vi "ManualControlL0SumnAdd.vi"(11 "Instrument VISA in":T1={"AWG VISA"="generadorpulsos", "Oscilloscope  VISA "="Oscilloscope", "Integration Board IP"="172.16.7.43", "connection ID"=refnum, "report out"=refnum, "report file path"=path "C:/Documents and Settings/CTA_LAB01/Desktop/L0_Asic/L0 Asic Test Data"}) -> (0 "error out":errorcluster, 3 "Instrument VISA out":T1={"AWG VISA"="generadorpulsos", "Oscilloscope  VISA "="Oscilloscope", "Integration Board IP"="172.16.7.43", "connection ID"=refnum, "report out"=refnum, "report file path"=path "C:/Documents and Settings/CTA_LAB01/Desktop/L0_Asic/L0 Asic Test Data"})   [LabVIEW 2009]
uses:
  <vilib>/Utility/NIReport.llb/NI_report.lvclass
  <vilib>/Utility/NIReport.llb/HTML/NI_HTML.lvclass
  Sum_Abrilader/L0_Sum_Adder Folder/C/Program Files/National Instruments/LabVIEW 2012/instr.lib/Agilent 8000 Series/Public/Configure/Configure Math (Binary Operation).vi
  Sum_Abrilader/L0_Sum_Adder Folder/C/Program Files/National Instruments/LabVIEW 2012/instr.lib/Agilent 8000 Series/Agilent 8000 Series.lvlib
panel:
  in  "error in (no error)":errorcluster
  in  "stop":bool
  in  "Enable 6":bool=TRUE
  in  "Enable 4":bool=TRUE
  in  "Enable 5":bool=TRUE
  in  "Enable 2":bool=TRUE
  in  "Enable 3":bool=TRUE
  in  "Enable 0":bool=TRUE
  in  "Enable 1":bool=TRUE
  in  "Amplitude":dbl=0.1 min=0.05 max=1.0 step=0.05
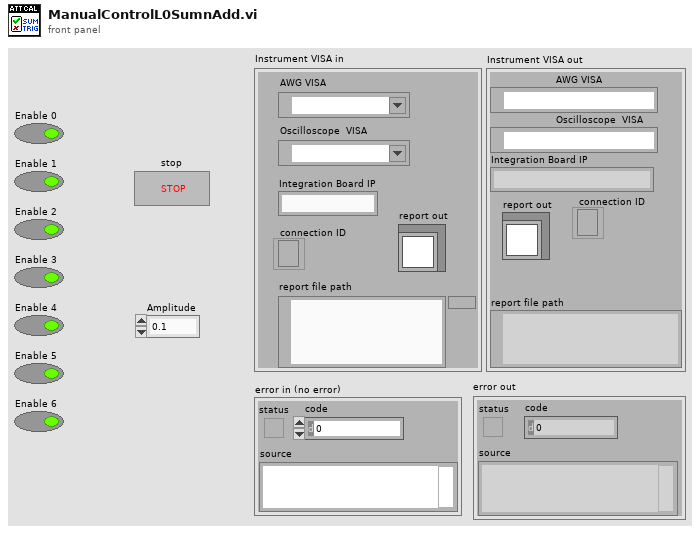
[diagram p1: front panel]
types:
  T1 = cluster{"AWG VISA":refnum<visa-resource-name>, "Oscilloscope  VISA ":refnum<visa-resource-name>, "Integration Board IP":string, "connection ID":refnum<k5>, "report out":refnum<class "NI_report.lvclass">, "report file path":path}
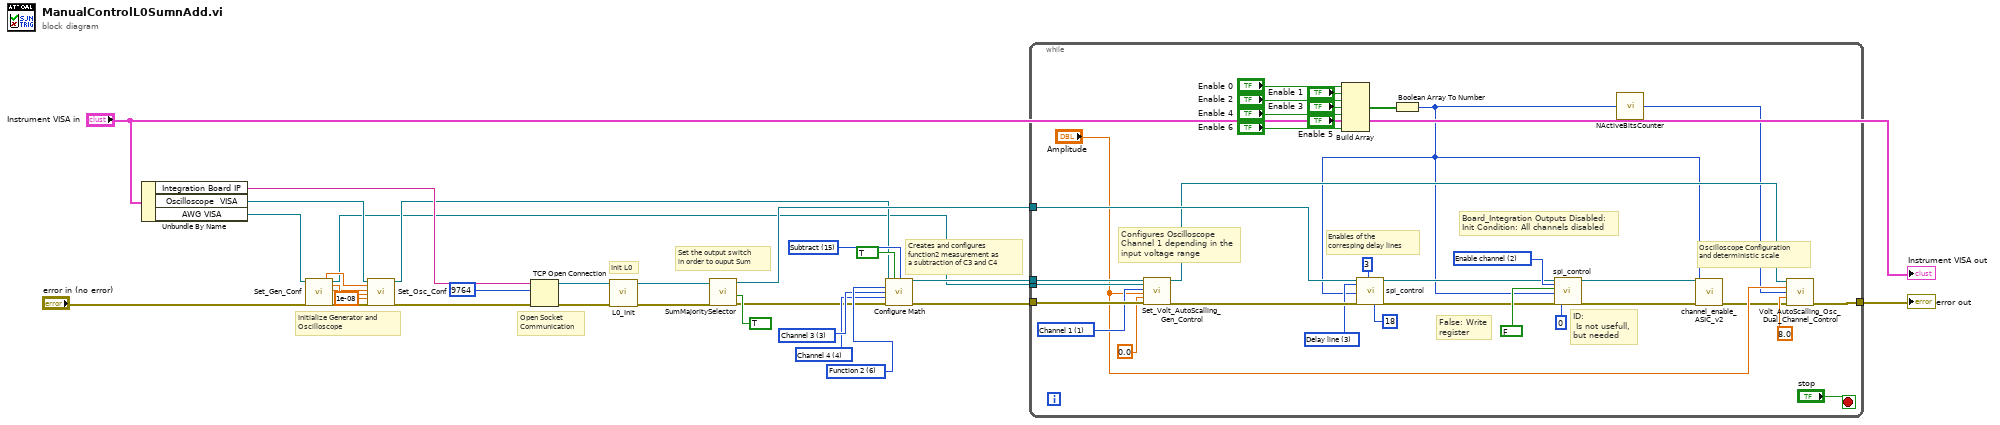
[diagram p0: block diagram]
diagram:
  w26 = u16 6 items=["Function 1"=5, "Function 2"=6, "Function 3"=7, "Function 4"=8] ("Math Channel (5: Function 1)")
  w27 = u16 15 items=["Add"=12, "Divide"=13, "Multiply"=14, "Subtract"=15, "Common Mode"=16, "Versus"=17] ("Math Operation (12: Add)")
  w25 = 3 items=["Channel 1"=1, "Channel 2"=2, "Channel 3"=3, "Channel 4"=4] ("Channel (1: Channel 1)")
  w24 = 4 items=["Channel 1"=1, "Channel 2"=2, "Channel 3"=3, "Channel 4"=4] ("Channel (1: Channel 1)")
  # "Initialize Generator and \nOscilloscope"
  # "Init L0"
  # "Creates and configures\nfunction2 measurement as\na subtraction of C3 and C4"
  # "Set the output switch\nin order to ouput Sum"
  # "Open Socket\nCommunication"
  n1 = Unbundle By Name("Instrument VISA in") -> ("Integration Board IP"=w18:string, "Oscilloscope  VISA"=w4:refnum<visa-resource-name>, "AWG VISA"=w5:refnum<visa-resource-name>)
  n2 = call "Set_Gen_Conf.vi"("AWG VISA"=w5, "error in (no error)"="error in (no error)") -> ("Amplitude 1 OUT"=w10:dbl, "VISA resource name out"=w2:refnum<visa-resource-name>, "Pulse Width in seconds 1 OUT"=w9:dbl, "Trigger Level 1"=w8:dbl, "error out"=w11:errorcluster)  [unwired: 10 in, 3 out]
  n3 = call "Set_Osc_Conf.vi"("VISA resource name"=w4, "Amplitude IN"=w10, "Trigger Level IN"=w8, "Pulse Width in seconds IN"=w9, "Position 1"=1e-08, "error in (no error)"=w11) -> ("VISA resource name out"=w3:refnum<visa-resource-name>, "error out"=w6:errorcluster)  [unwired: 12 in]
  n4 = TCP Open Connection(address=w18, remote port or service name=u16 9764, error in (no error)=w6) -> (connection ID=w16:refnum<k5>, error out=w15:errorcluster)  [unwired: 2 in]
  n5 = call "L0_Init.vi"("error in"=w15, "connection ID in"=w16) -> ("error out"=w13:errorcluster, "connection ID out"=w14:refnum<k5>)  [unwired: 8 in]
  n6 = call "SumMajoritySelector.vi"("On Sum\nOff Majority"=TRUE ("On Sum\nOff Majority"), "error in (no error)"=w13, "connection ID"=w14) -> ("error out"=w20:errorcluster, "connection ID out"=w21:refnum<k5>)  [unwired: 5 in]
  n7 = call-poly "Configure Math.vi"("VISA resource name"=w3, "Enable Math Channel (T:Enable)"=TRUE, "Math Operation (12: Add)"=w27, "Math Channel (5: Function 1)"=w26, "Math Operand (1: Channel 1)"=w25, "Math Operand (2: Channel 2)"=w24, "error in (no error)"=w20) -> ("VISA resource name out"=w12:refnum<visa-resource-name>, "error out"=w23:errorcluster)  [unwired: 7 in]
  n8 = while {
    tunnel: w21 -> [w57]
    tunnel: w23 -> [w62]
    tunnel: w2 -> [w59]
    tunnel: w12 -> [w58]
    tunnel: [w40] -> w19
    stop <- "stop" stop-if-true
    w47 = u16 2 items=["Attenuation", "Clipping", "Enable channel", "Delay line", "ASIC"] ("Device")
    w50 = u16 3 items=["Attenuation", "Clipping", "Enable channel", "Delay line", "ASIC"] ("Device")
    w61 = 1 items=["Channel 1"=1, "Channel 2"=2, "Channel 3"=3, "Channel 4"=4] ("Channel")
    # "Enables of the\ncorresping delay lines"
    # "False: Write\nregister"
    # "ID:\n Is not usefull, \nbut needed"
    # "Board_Integration Outputs Disabled:\nInit Condition: All channels disabled"
    # "Oscilloscope Configuration \nand deterministic scale"
    # "Configures Oscilloscope\nChannel 1 depending in the \ninput voltage range"
    n9 = call "Set_Volt_AutoScalling_Gen_Control.vi"("VISA Oscilloscope"=w58, "VISA Generator"=w59, "Channel"=w61, "Amplitude"="Amplitude", "DC Offset"=0.0, "error in (no error)"=w62) -> ("VISA Oscilloscope"=w55:refnum<visa-resource-name>, "error out"=w56:errorcluster)  [unwired: 11 in, 1 out]
    n10 = Build Array("Enable 0", "Enable 1", "Enable 2", "Enable 3", "Enable 4", "Enable 5", "Enable 6") -> (w39:bool[])
    n11 = Boolean Array To Number(Boolean array=w39) -> (number=w31:u32)
    n12 = call "spi_control.vi"("connection ID"=w57, "Device"=w50, "Data"=w31, "Register or channel"=18, "error out 3"=w56, "chip delay"=3) -> ("connection ID out"=w45:refnum<k5>, "error out 2"=w44:errorcluster)  [unwired: 6 in, 6 out]
    n13 = call "spi_control.vi"("connection ID"=w45, "Device"=w47, "Read/#write"=FALSE, "Data"=w31, "error out 3"=w44, "Id in"=0) -> ("connection ID out"=w43:refnum<k5>, "error out 2"=w42:errorcluster)  [unwired: 6 in, 6 out]
    n14 = call "NActiveBitsCounter.vi"("Input Number"=w31) -> ("N High Bits"=w41:i32)
    n15 = call "channel_enable_ASIC_v2.vi"("error in"=w42, "Channel Combination"=w31, "Connection ID in"=w43) -> ("error out"=w49:errorcluster)  [unwired: 7 in, 1 out]
    n16 = call "Volt_AutoScalling_Osc_Dual_Channel_Control.vi"("VISA Oscilloscope"=w55, "Voltage In"="Amplitude", "N Channels"=w41, "Offset Divider"=8.0, "error in"=w49) -> ("error out"=w40:errorcluster)  [unwired: 9 in, 1 out]
  }
  "error out" <- w19
  "Instrument VISA out" <- "Instrument VISA in"
